vi "Set Conn Pane Recommended to Required.vi"(8 "error in (no error)":errorcluster, 10 "Save VI (T)":bool=TRUE, 11 "vi path":path) -> (0 "error out":errorcluster)   [LabVIEW 2023]
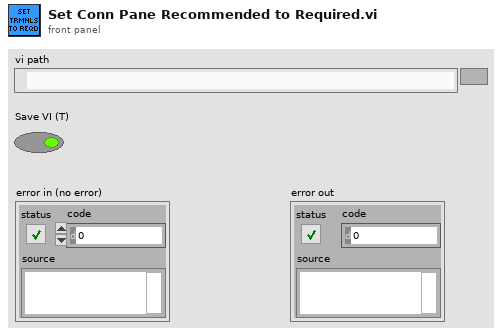
[diagram p1: front panel]
types:
  T1 = enum16{"Invalid Wire Rule", "Required", "Recommended", "Optional", "Dynamic Dispatch"}[]
  T2 = enum16{"Invalid Wire Rule", "Required", "Recommended", "Optional", "Dynamic Dispatch"}
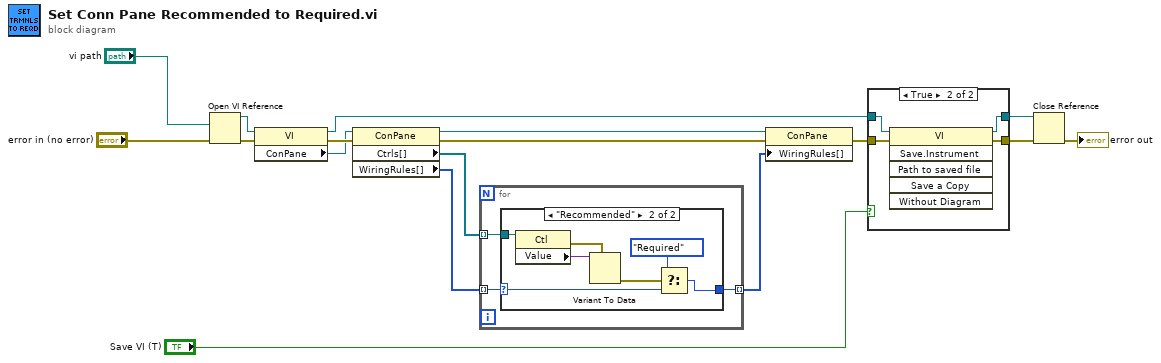
[diagram p0: block diagram]
diagram:
  n1 = Open VI Reference(vi path="vi path", error in (no error)="error in (no error)") -> (vi reference=w16:refnum<vi>, error out=w15:errorcluster)  [unwired: 4 in]
  n2 = property class="VI"(reference=w16, error in=w15) -> (reference out=w3:refnum<vi>, error out=w14:errorcluster, "ConPane"=w1:refnum<vi>)
  n3 = property class="ConPane"(reference=w1, error in=w14) -> (reference out=w11:refnum<vi>, error out=w12:errorcluster, "Ctrls[]"=w2:refnum<vi>[], "WiringRules[]"=w13:T1)
  n4 = for {
    tunnel: w13 -> [w20] mode=indexing
    tunnel: [w19] -> w10 mode=indexing
    tunnel: w2 -> [w18] mode=indexing
    n5 = case shown="\"Recommended\"" w20 {
      selector: w20 -> [w21 w24]
      tunnel: [w21 w23] -> w19
      tunnel: w18 -> [_ w22]
      frame Default {
      }
      frame "Recommended" {
        n6 = property class="Ctl"(reference=w22) -> (error out=w27:errorcluster, "Value"=w28:variant)  [unwired: 1 in, 1 out]
        n7 = Variant To Data(type=w27, Variant=w28) -> (error out=w26:errorcluster)  [unwired: 1 in, 1 out]
        n8 = Select(t=T2."Required" ("Wire Rule"), s=w26, f=w24) -> (s? t:f=w23:T2)
      }
    }
  }
  n9 = property class="ConPane"(reference=w11, error in=w12, "WiringRules[]"=w10) -> (error out=w7:errorcluster)  [unwired: 1 out]
  n10 = case shown="True" "Save VI (T)" {
    tunnel: w7 -> [w30 w34]
    tunnel: [w30 w33] -> w6
    tunnel: [w29 w32] -> w5
    tunnel: w3 -> [w29 w31]
    frame False {
    }
    frame True {
      n11 = invoke class="VI" method="Save.Instrument"(reference=w31, error in=w34) -> (reference out=w32:refnum<vi>, error out=w33:errorcluster)  [unwired: 4 in, 4 out]
    }
  }
  n12 = Close Reference(reference=w5, error in (no error)=w6) -> (error out=→"error out":errorcluster)
